vi "CreateReports.vi"(8 "error in (no error)":errorcluster, 11 "S1 in":refnum<class "S4.lvclass">) -> (0 "error out":errorcluster, 3 "S1 out":refnum<class "S4.lvclass">)   [LabVIEW 2018, in "S4.lvclass"]
uses:
  S4.lvclass
  <vilib>/Utility/sysdir.llb/System Directory Type.ctl
  S4.lvclass/S4.ctl
  <vilib>/Utility/file.llb/Write Delimited Spreadsheet (string).vi
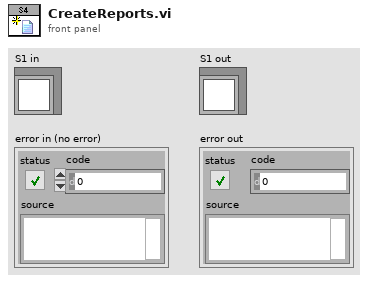
[diagram p1: front panel]
types:
  T1 = typedef "System Directory Type.ctl" = i32
  T2 = enum16{"open", "replace", "create", "open or create", "replace or create", "replace or create with confirmation"}
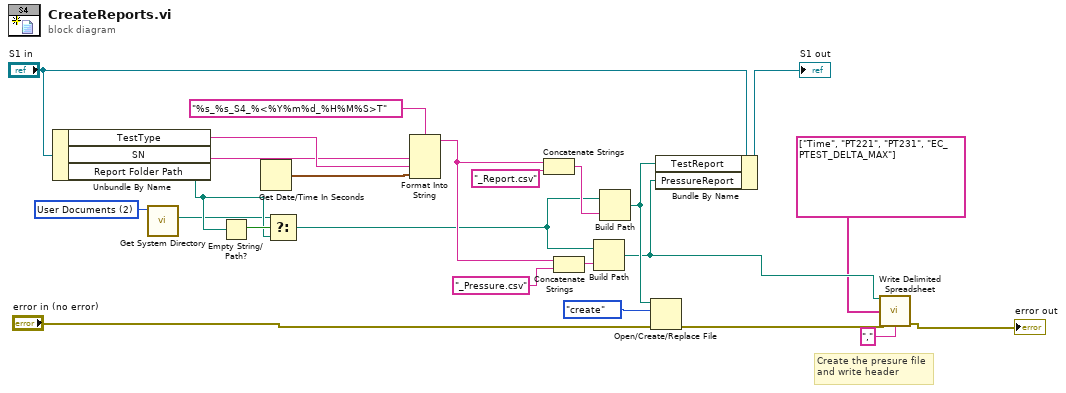
[diagram p0: block diagram]
diagram:
  w2 = T1 2 items=["User Home"=0, "User Desktop"=1, "User Documents"=2, "User Application Data"=3, "User Preferences"=4, "User Temporary"=5, "Public Documents"=6, "Public Application Data"=7, "Public Preferences"=8, "Public Cache"=13, "System Core Libraries"=9, "System Installed Libraries"=10, "Application Files"=11, "Boot Volume Root"=12] ("system directory type")
  # "Create the presure file\nand write header"
  n1 = Unbundle By Name("S1 in") -> ("TestType"=w15:string, "SN"=w14:string, "Report Folder Path"=w4:path)
  n2 = call <vilib>:"Get System Directory.vi"("system directory type"=w2) -> ("system directory"=w1:path)  [unwired: 10 in]
  n3 = Empty String/Path?(string/path=w4) -> (empty?=w5:bool)
  n4 = Get Date/Time In Seconds() -> (seconds since 1Jan1904=w16:timestamp)
  n5 = Select(t=w1, s=w5, f=w4) -> (s? t:f=w3:path)
  n6 = Format Into String(format string="%s_%s_S4_%<%Y%m%d_%H%M%S>T", w14, w15, w16) -> (resulting string=w18:string)  [unwired: 2 in, 1 out]
  n7 = Concatenate Strings(w18, "_Report.csv" ("string")) -> (w20:string)
  n8 = Concatenate Strings(w18, "_Pressure.csv" ("string")) -> (w22:string)
  n9 = Build Path(base path=w3, name or relative path=w22) -> (appended path=w10:path)
  n10 = Build Path(base path=w3, name or relative path=w20) -> (appended path=w24:path)
  n11 = Open/Create/Replace File(file path (use dialog)=w24, error in="error in (no error)", operation (0:open)=T2."create") -> (error out=w9:errorcluster)  [unwired: 3 in, 2 out]
  n12 = Bundle By Name(cluster="S1 in", "TestReport"=w24, "PressureReport"=w10) -> (→"S1 out":refnum<class "S4.lvclass">)
  n13 = call-poly <vilib>:"Write Delimited Spreadsheet.vi"("file path (dialog if empty)"=w10, "1D data"=string[] ["Time", "PT221", "PT231", "EC_PTEST_DELTA_MAX"], "error in (no error)"=w9, "delimiter (\\t)"="," ("delimiter (\\t)")) -> ("error out"=→"error out":errorcluster)  [unwired: 10 in, 1 out]
